vi "Transform1ToDiff.vi"(2 "Transform":T1) -> (0 "Differential Motion Vector":dbl[](array[numeric]))   [LabVIEW 2017, in "NI_Kinematics.lvlib"]
uses:
  <vilib>/robotics/Kinematics/NI_Kinematics.lvlib
  <vilib>/Analysis/Matrix/Datatypes/RealMatrix.ctl
  <vilib>/Analysis/Matrix/NI_Matrix.lvlib
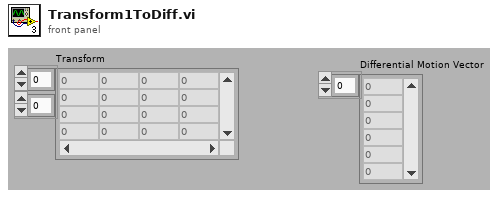
[diagram p1: front panel]
types:
  T1 = typedef "NI_Matrix.lvlib/RealMatrix.ctl" = dbl[][]
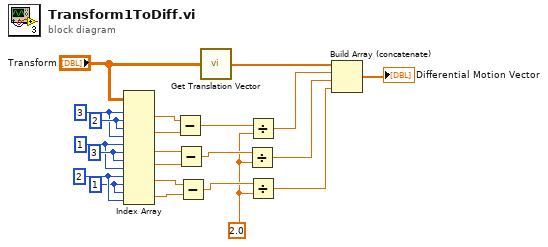
[diagram p0: block diagram]
diagram:
  w1 = 2.0
  w15 = 1 ("index (row)")
  w16 = 2 ("index (row)")
  w18 = 3 ("index (row)")
  w17 = 1 ("index (row)")
  w20 = 2 ("index (row)")
  w19 = 3 ("index (row)")
  n1 = Index Array(array="Transform", index (row) #1=w19, index (col) #1=w20, index (row) #2=w20, index (col) #2=w19, index (row) #3=w17, index (col) #3=w18, index (row) #4=w18, index (col) #4=w17, index (row) #5=w16, index (col) #5=w15, index (row) #6=w15, index (col) #6=w16) -> (element #1=w14:dbl, element #2=w13:dbl, element #3=w12:dbl, element #4=w11:dbl, element #5=w10:dbl, element #6=w9:dbl)
  n2 = Subtract(x=w14, y=w13) -> (x-y=w4:dbl)
  n3 = Subtract(x=w12, y=w11) -> (x-y=w3:dbl)
  n4 = Subtract(x=w10, y=w9) -> (x-y=w2:dbl)
  n5 = call <vilib>:"Get Translation Vector.vi"("transform"="Transform") -> ("translation vector"=w22:dbl[])
  n6 = Divide(x=w3, y=w1) -> (x/y=w6:dbl)
  n7 = Divide(x=w4, y=w1) -> (x/y=w5:dbl)
  n8 = Divide(x=w2, y=w1) -> (x/y=w7:dbl)
  n9 = Build Array (concatenate)(w22, w5, w6, w7) -> (→"Differential Motion Vector":dbl[])
